vi "indicators+variable resestors.vi"() -> ()   [LabVIEW 2017]
panel:
  out "Boolean 2":bool
  out "Boolean":bool
  in  "Knob 2":dbl(knob) scale=0.0..12.0
  in  "Knob":dbl(knob) scale=0.0..12.0
  out "Gauge":cluster{dbl, dbl}(knob) scale=0.0..12.0
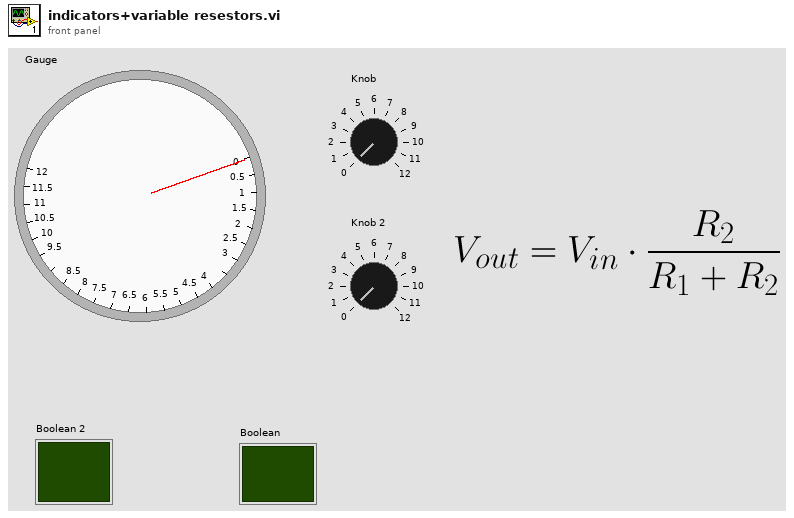
[diagram p1: front panel]
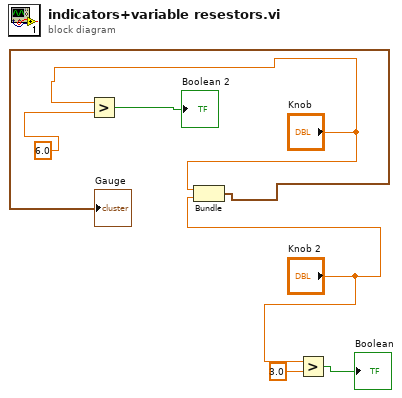
[diagram p0: block diagram]
diagram:
  n1 = Greater?(x="Knob", y=6.0 ("x")) -> (0:→"Boolean 2":bool)
  n2 = Bundle("Knob"="Knob", "Knob 2"="Knob 2") -> (→"Gauge":cluster{"Knob":dbl, "Knob 2":dbl})  [unwired: 1 in]
  n3 = Greater?(x="Knob 2", y=3.0) -> (0:→"Boolean":bool)
